vi "Configure Reference Levels [WM] Core.vi"(0 "CS++Scope":refnum<class "CS++Scope.lvclass">, 5 "low reference (10.0%)":dbl=10.0 format="%.3f", 7 "mid reference (50.0%)":dbl=50.0 format="%.3f", 9 "high reference (90.0%)":dbl=90.0 format="%.3f", 11 "error in (no error)":errorcluster) -> (4 "CS++Scope out":refnum<class "CS++Scope.lvclass">, 15 "error out":errorcluster)   [LabVIEW 2015, in "CS++Scope.lvlib" / "CS++Scope.lvclass"]
doc: "This VI configures the reference levels for waveform measurements. \n\nYou must call this VI before you call the IviScope Read Waveform Measurement [WM] or IviScope Fetch Waveform Measurement [WM] to take a rise time, fall time, width negative, width positive, duty cycle negative, duty cycle positive, preshoot, or overshoot measurement.\n\nNotes:\n\n(1) This VI is part of the IviScopeWaveformMeasurement [WM] extension group."
uses:
  CS++Scope.lvclass
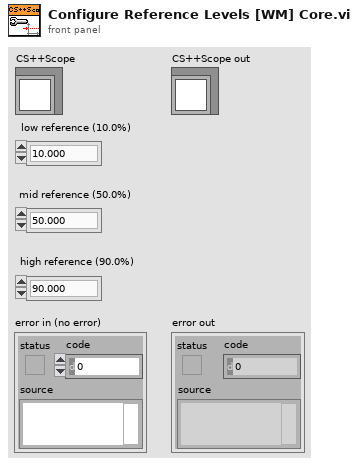
[diagram p1: front panel]
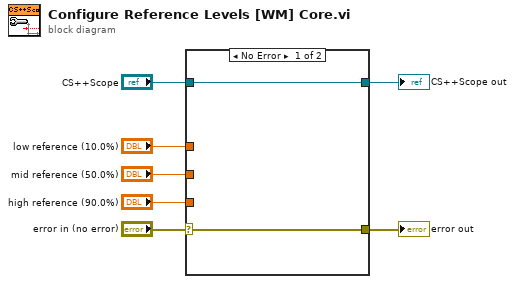
[diagram p0: block diagram]
diagram:
  n1 = case shown="No Error" "error in (no error)" {
    selector: "error in (no error)" -> [w8 w11]
    tunnel: [w8 w11] -> w6
    tunnel: [w9 w10] -> w2
    tunnel: "CS++Scope" -> [w9 w10]
    tunnel: "low reference (10.0%)" -> [_ _]
    tunnel: "mid reference (50.0%)" -> [_ _]
    tunnel: "high reference (90.0%)" -> [_ _]
    frame No Error {
    }
    frame Error {
    }
  }
  "error out" <- w6
  "CS++Scope out" <- w2
